vi "K-F (SubVI).vi"(11 "Град K":dbl) -> (3 "Град F":dbl)   [LabVIEW 2020]
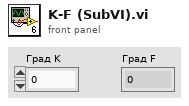
[diagram p1: front panel]
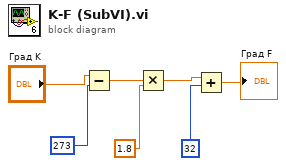
[diagram p0: block diagram]
diagram:
  n1 = Subtract(x="Град K", y=273) -> (x-y=w3:dbl)
  n2 = Multiply(x=w3, y=1.8) -> (x*y=w5:dbl)
  n3 = Add(x=w5, y=32) -> (x+y=→"Град F":dbl)
